vi "Read Attributes.vi"(11 "Set PCC Transition Msg":refnum<class "Set PCC Transition Msg.lvclass">) -> (2 "Payload":cluster{"PCC_Transition":T1})   [LabVIEW 2018, in "Device Communication and Control Abstract Actor.lvlib" / "Set PCC Transition Msg.lvclass"]
uses:
  Set PCC Transition Msg.lvclass
  <vilib>/ORNL/CSEISMIC DDS/CSEISMIC DDS Base/Data Types/PCC_Transition.ctl
  <vilib>/ORNL/CSEISMIC DDS/CSEISMIC DDS Base/Data Types/Controls/DeviceID.ctl
  Set PCC Transition Msg.lvclass/Set PCC Transition Msg.ctl
  <vilib>/ORNL/CSEISMIC DDS/CSEISMIC DDS Base/CSEISMIC DDS.lvclass
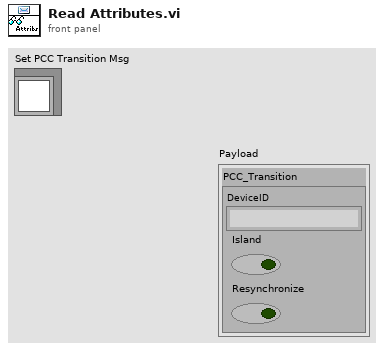
[diagram p1: front panel]
types:
  T1 = typedef "CSEISMIC DDS.lvlib/CSEISMIC DDS.lvclass/PCC_Transition.ctl" = cluster{"DeviceID":T2, "Island":bool, "Resynchronize":bool}
  T2 = typedef "CSEISMIC DDS.lvlib/CSEISMIC DDS.lvclass/DeviceID.ctl" = string
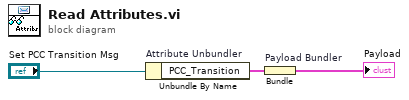
[diagram p0: block diagram]
diagram:
  n1 = Unbundle By Name "Attribute Unbundler"("Set PCC Transition Msg") -> ("PCC_Transition"=w1:T1)
  n2 = Bundle "Payload Bundler"("PCC_Transition"=w1) -> (→"Payload":cluster{"PCC_Transition":T1})  [unwired: 1 in]
